vi "Set Wire Label Visible.vi"(8 "error in (no error)":errorcluster, 10 "Connected Wire.Label.Visible":bool, 11 "CSM-Helper in":refnum<class "CSM-Helper.lvclass">) -> (0 "error out":errorcluster, 3 "CSM-Helper out":refnum<class "CSM-Helper.lvclass">)   [LabVIEW 2017, in "CSM-Helper.lvclass"]
doc: "### Set Wire Label Visible.vi\n\n-- <b>Controls</b> --\n- <b>Connected Wire.Label.Visible</b>:\n- <b>CSM-Helper in</b>: CSMHelper input\n\n-- <b>Indicators</b> --\n- <b>CSM-Helper out</b>: CSMHelper output"
uses:
  CSM-Helper.lvclass
  CSM-Helper.lvclass/CSM-Helper.ctl
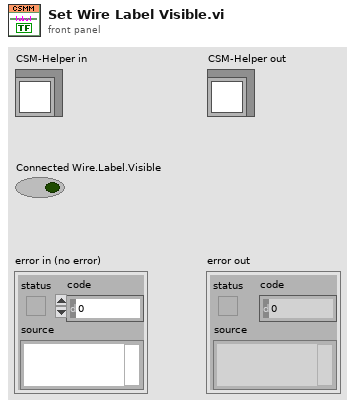
[diagram p1: front panel]
types:
  T1 = typedef "CSM-Helper.lvclass/_csmhelper_Front_Tunnels_Refs.ctl" = cluster{"Registration":refnum<vi>, "InternalData":refnum<vi>, "CSM Name":refnum<vi>, "Last Resp":refnum<vi>, "Remaining State":refnum<vi>, "Arguments":refnum<vi>, "Response Source":refnum<vi>, "Source CSM":refnum<vi>, "Selector":refnum<vi>, "Error":refnum<vi>}
  T2 = typedef "CSM-Helper.lvclass/_csmhelper_Back_Tunnels_Refs.ctl" = cluster{"Registration":refnum<vi>, "InternalData":refnum<vi>, "Resp":refnum<vi>, "Remaining State":refnum<vi>, "Error":refnum<vi>}
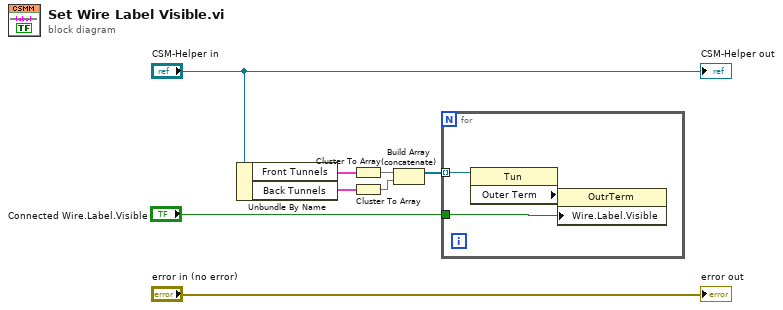
[diagram p0: block diagram]
diagram:
  n1 = Unbundle By Name("CSM-Helper in") -> ("Front Tunnels"=w4:T1, "Back Tunnels"=w3:T2)
  n2 = Cluster To Array(cluster=w4) -> (array=w6:refnum<vi>[])
  n3 = Cluster To Array(cluster=w3) -> (array=w1:refnum<vi>[])
  n4 = Build Array (concatenate)(w6, w1) -> (w2:refnum<vi>[])
  n5 = for {
    tunnel: w2 -> [w11] mode=indexing
    tunnel: "Connected Wire.Label.Visible" -> [w9]
    n6 = property class="Tun"(reference=w11) -> ("Outer Term"=w10:refnum<vi>)  [unwired: 1 in, 2 out]
    n7 = property class="OutrTerm"(reference=w10, "Wire.Label.Visible"=w9) -> ()  [unwired: 1 in, 2 out]
  }
  "error out" <- "error in (no error)"
  "CSM-Helper out" <- "CSM-Helper in"
